vi "spec_getCalibration.vi"(8 "error in (no error)":errorcluster, 11 "LightField Automation in":refnum<class "LightField Automation.lvclass">) -> (0 "error out":errorcluster, 2 "ColumnCalibration":dbl[](array[numeric]), 3 "LightField Automation out":refnum<class "LightField Automation.lvclass">)   [LabVIEW 2020, in "LightField Automation.lvclass"]
uses:
  LightField Automation.lvclass
  LightField Automation.lvclass/LightField Automation.ctl
  C:/Program Files/Princeton Instruments/LightField/AddInViews/PrincetonInstruments.LightFieldViewV3.dll
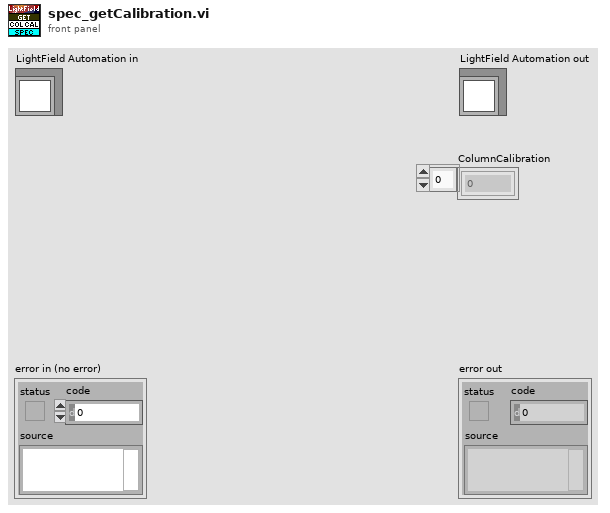
[diagram p1: front panel]
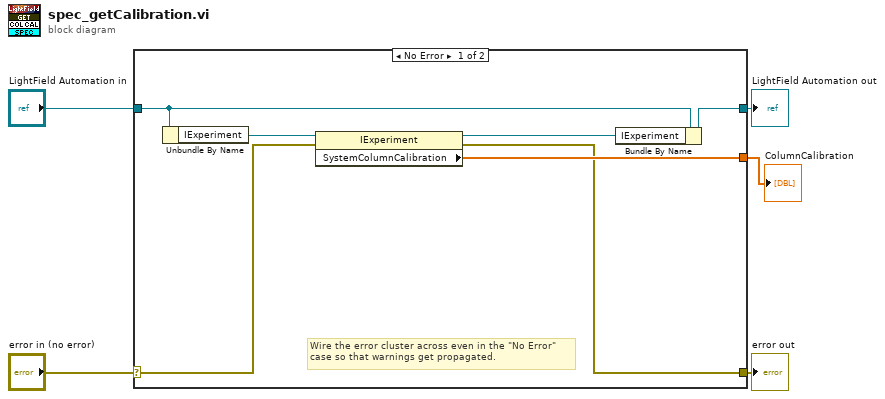
[diagram p0: block diagram]
diagram:
  n1 = case shown="No Error" "error in (no error)" {
    selector: "error in (no error)" -> [w10 w14]
    tunnel: [w9 w14] -> w4
    tunnel: [w7 w13] -> w2
    tunnel: "LightField Automation in" -> [w8 w13]
    tunnel: [w11 _] -> w1
    frame No Error {
      # "Wire the error cluster across even in the \"No Error\"\ncase so that warnings get propagated."
      n2 = Unbundle By Name(w8) -> ("IExperiment"=w12:refnum<k24>)
      n3 = property class="IExperiment"(reference=w12, error in=w10) -> (reference out=w6:refnum<k24>, error out=w9:errorcluster, "SystemColumnCalibration"=w11:dbl[])
      n4 = Bundle By Name(cluster=w8, "IExperiment"=w6) -> (w7:refnum<class "LightField Automation.lvclass">)
    }
    frame Error {
    }
  }
  "error out" <- w4
  "LightField Automation out" <- w2
  "ColumnCalibration" <- w1
